vi "Heartbeat check.vi"(8 "error in":errorcluster, 11 "CANopen in":refnum<class "CANopen.lvclass">) -> (0 "error out":errorcluster, 2 "Emergency":bool, 3 "CANopen out":refnum<class "CANopen.lvclass">)   [LabVIEW 2026, in "canopen_.lvlib" / "CANopen.lvclass"]
doc: "Checks for watchdogs alarm in the heartbeat table. If a watchdog has elapsed, the error cluster is set accordingly."
uses:
  CANopen.lvclass
  CANopen.lvclass/CANopen.ctl
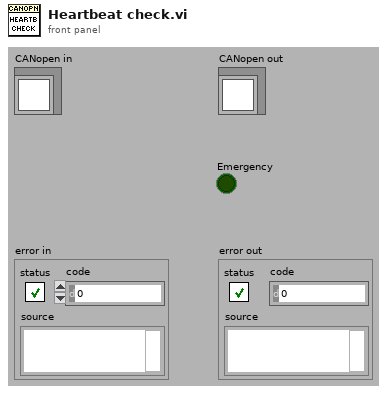
[diagram p1: front panel]
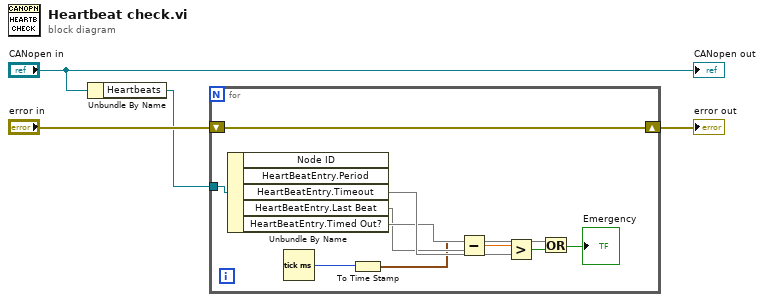
[diagram p0: block diagram]
diagram:
  n1 = Unbundle By Name("CANopen in") -> ("Heartbeats"=w1:refnum<data-value>)
  n2 = for {
    tunnel: w1 -> [w14]
    shift-right: [w13] -> w2
    shift-left: "error in" -> [w13]
    n3 = Unbundle By Name(w14) -> ("HeartBeatEntry.Timeout"=w11, "HeartBeatEntry.Last Beat"=w7, "HeartBeatEntry.Timed Out?"=w8)  [unwired: 2 out]
    n4 = Tick Count (ms)() -> (millisecond timer value=w6:u32)
    n5 = To Time Stamp(1:w6) -> (0:w5:timestamp)
    n6 = Subtract(x=w5, y=w7) -> (x-y=w12:dbl)
    n7 = Greater?(x=w12, y=w11) -> (0:w10:bool)
    n8 = Or(x=w8, y=w10) -> (x .or. y?=→"Emergency":bool)
  }
  "error out" <- w2
  "CANopen out" <- "CANopen in"
